vi "writeread_timestamp.vi"(0 "VISA resource input":refnum<visa-resource-name>, 1 "Read Delay":dbl, 2 "write buffer":string, 3 "error in (no error)":errorcluster) -> (6 "VISA resource out":refnum<visa-resource-name>, 7 "Response 2":string, 9 "error out":errorcluster)   [LabVIEW 2018]
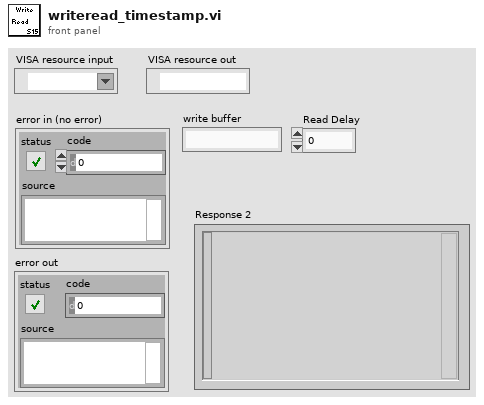
[diagram p1: front panel]
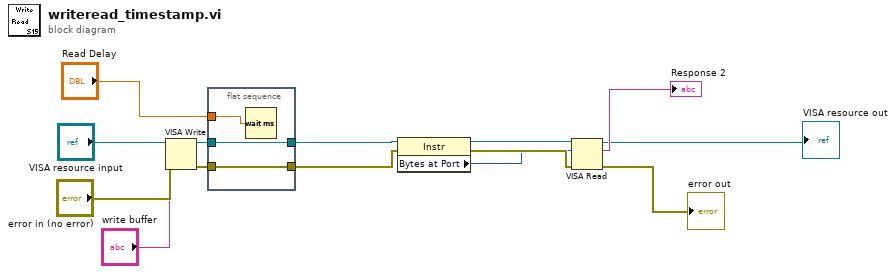
[diagram p0: block diagram]
diagram:
  n1 = VISA Write(VISA resource name="VISA resource input", write buffer="write buffer", error in (no error)="error in (no error)") -> (VISA resource name out=w13:refnum<visa-resource-name>, error out=w14:errorcluster)  [unwired: 1 out]
  n2 = flat-sequence {
    tunnel: w14 -> [w16]
    tunnel: [w16] -> w2
    tunnel: w13 -> [w15]
    tunnel: [w15] -> w5
    tunnel: "Read Delay" -> [w17]
    frame #0 {
      n3 = Wait (ms)(milliseconds to wait=w17) -> ()  [unwired: 1 out]
    }
  }
  n4 = property class="Instr"(reference=w5, error in=w2) -> (reference out=w4:refnum<visa-resource-name>, error out=w3:errorcluster, "Bytes at Port"=w1:u32)
  n5 = VISA Read(VISA resource name=w4, byte count=w1, error in (no error)=w3) -> (VISA resource name out=→"VISA resource out":refnum<visa-resource-name>, read buffer=→"Response 2":string, error out=→"error out":errorcluster)  [unwired: 1 out]
